vi "Read CtlRef.vi"(8 "error in (no error)":errorcluster, 11 "ControlDragStartingMsg In":refnum<class "ControlDragStartingMsg.lvclass">) -> (0 "error out":errorcluster, 2 "CtlRef":refnum<vi>, 3 "ControlDragStartingMsg Out":refnum<class "ControlDragStartingMsg.lvclass">)   [LabVIEW 2018, in "MVA Framework.lvlib" / "ActorEvents.lvlib" / "ControlDragStartingMsg.lvclass"]
uses:
  ControlDragStartingMsg.lvclass
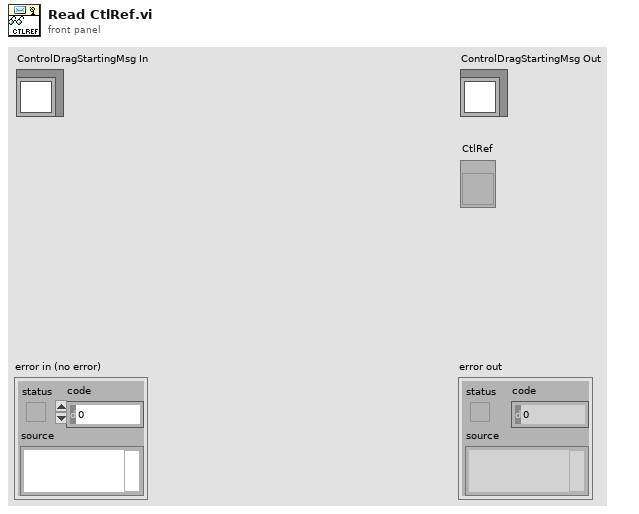
[diagram p1: front panel]
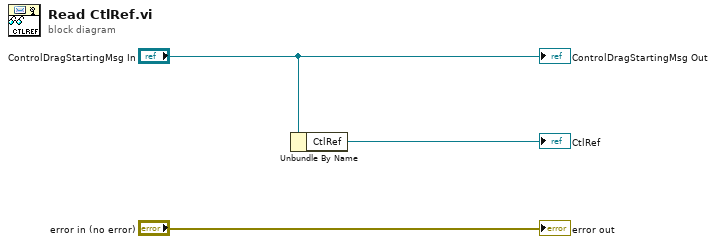
[diagram p0: block diagram]
diagram:
  n1 = Unbundle By Name("ControlDragStartingMsg In") -> ("CtlRef"=→"CtlRef":refnum<vi>)
  "error out" <- "error in (no error)"
  "ControlDragStartingMsg Out" <- "ControlDragStartingMsg In"
